vi "WiFiConnection.vi"(9 "Login":cluster{"SSID":string, "password":string}={"SSID"="SSID", "password"="password"}, 11 "Data In":T1) -> (3 "Data Out":T1={"Port"="", "All Code"="Hi"})   [LabVIEW 2016]
uses:
  uPythonX/PythonData.ctl
  uPythonX/uPythonX.xctl
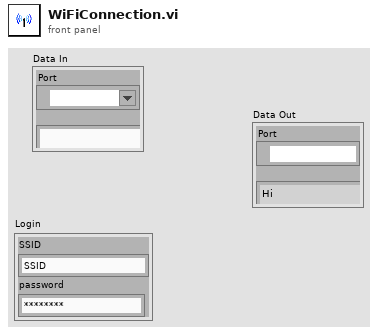
[diagram p1: front panel]
types:
  T1 = typedef "uPythonX.xctl/PythonData.ctl" = cluster{"Port":refnum<visa-resource-name>, "All Code":string}
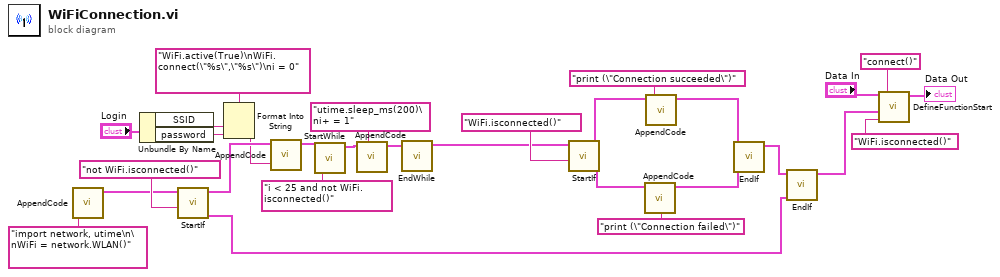
[diagram p0: block diagram]
diagram:
  n1 = call "AppendCode.vi"("New Code"="import network, utime\n\nWiFi = network.WLAN()") -> ("Data Out"=w26:T1)  [unwired: 10 in]
  n2 = Unbundle By Name("Login") -> ("SSID"=w22:string, "password"=w23:string)
  n3 = call "StartIf.vi"("Comparison"="not WiFi.isconnected()", "Data In"=w26) -> ("False Out"=w6:T1, "True Out"=w21:T1)  [unwired: 8 in]
  n4 = Format Into String(format string="WiFi.active(True)\nWiFi.connect(\"%s\",\"%s\")\ni = 0" ("New Code"), w22, w23) -> (resulting string=w20:string)  [unwired: 2 in, 1 out]
  n5 = call "AppendCode.vi"("New Code"=w20, "Data In"=w21) -> ("Data Out"=w9:T1)  [unwired: 9 in]
  n6 = call "StartWhile.vi"("Comparison"="i < 25 and not WiFi.isconnected()", "Data In"=w9) -> ("Data Out"=w18:T1)  [unwired: 9 in]
  n7 = call "AppendCode.vi"("New Code"="utime.sleep_ms(200)\ni+ = 1", "Data In"=w18) -> ("Data Out"=w7:T1)  [unwired: 9 in]
  n8 = call "EndWhile.vi"("Data In"=w7) -> ("Data Out"=w8:T1)  [unwired: 10 in]
  n9 = call "StartIf.vi"("Comparison"="WiFi.isconnected()", "Data In"=w8) -> ("False Out"=w14:T1, "True Out"=w15:T1)  [unwired: 8 in]
  n10 = call "AppendCode.vi"("New Code"="print (\"Connection failed\")", "Data In"=w14) -> ("Data Out"=w12:T1)  [unwired: 9 in]
  n11 = call "AppendCode.vi"("New Code"="print (\"Connection succeeded\")", "Data In"=w15) -> ("Data Out"=w13:T1)  [unwired: 9 in]
  n12 = call "EndIf.vi"("False In"=w12, "True In"=w13) -> ("Data Out"=w5:T1)  [unwired: 9 in]
  n13 = call "EndIf.vi"("False In"=w6, "True In"=w5) -> ("Data Out"=w3:T1)  [unwired: 9 in]
  n14 = call "DefineFunctionStart.vi"("Function name"="connect()", "return"="WiFi.isconnected()", "Function"=w3, "Data In"="Data In") -> ("Data Out"=→"Data Out":T1)  [unwired: 7 in]
